vi "Host Datalog.vi"(6 "Operation":enum16{"Create", "Write", "Close", "Header"}(ring)=enum."Write", 8 "error in":errorcluster, 10 "Enable":bool) -> (0 "error out":errorcluster, 5 "datalog Q":refnum<queue>)   [LabVIEW 2021]
doc: "Host data logging is done as four files as Power& Battery, Navigation and HSSS, Ballast and Thrusters, 50KWh battery. every one hour the new files will be created . The data for the vi will be accumulated from Update GUI through Queue"
uses:
  <vilib>/Utility/sysdir.llb/System Directory Type.ctl
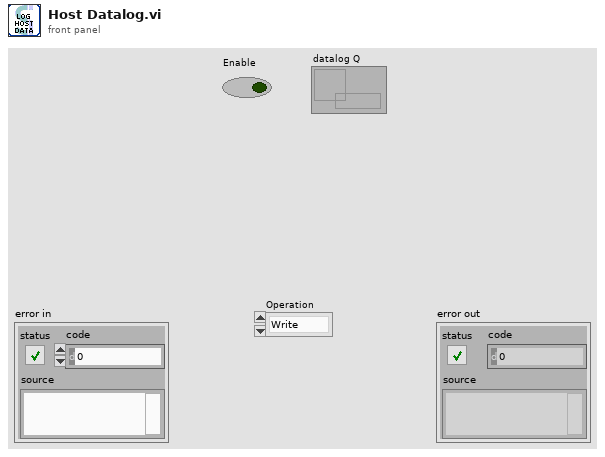
[diagram p1: front panel]
types:
  T1 = enum16{"open", "replace", "create", "open or create", "replace or create", "replace or create with confirmation"}
  T2 = typedef "System Directory Type.ctl" = i32
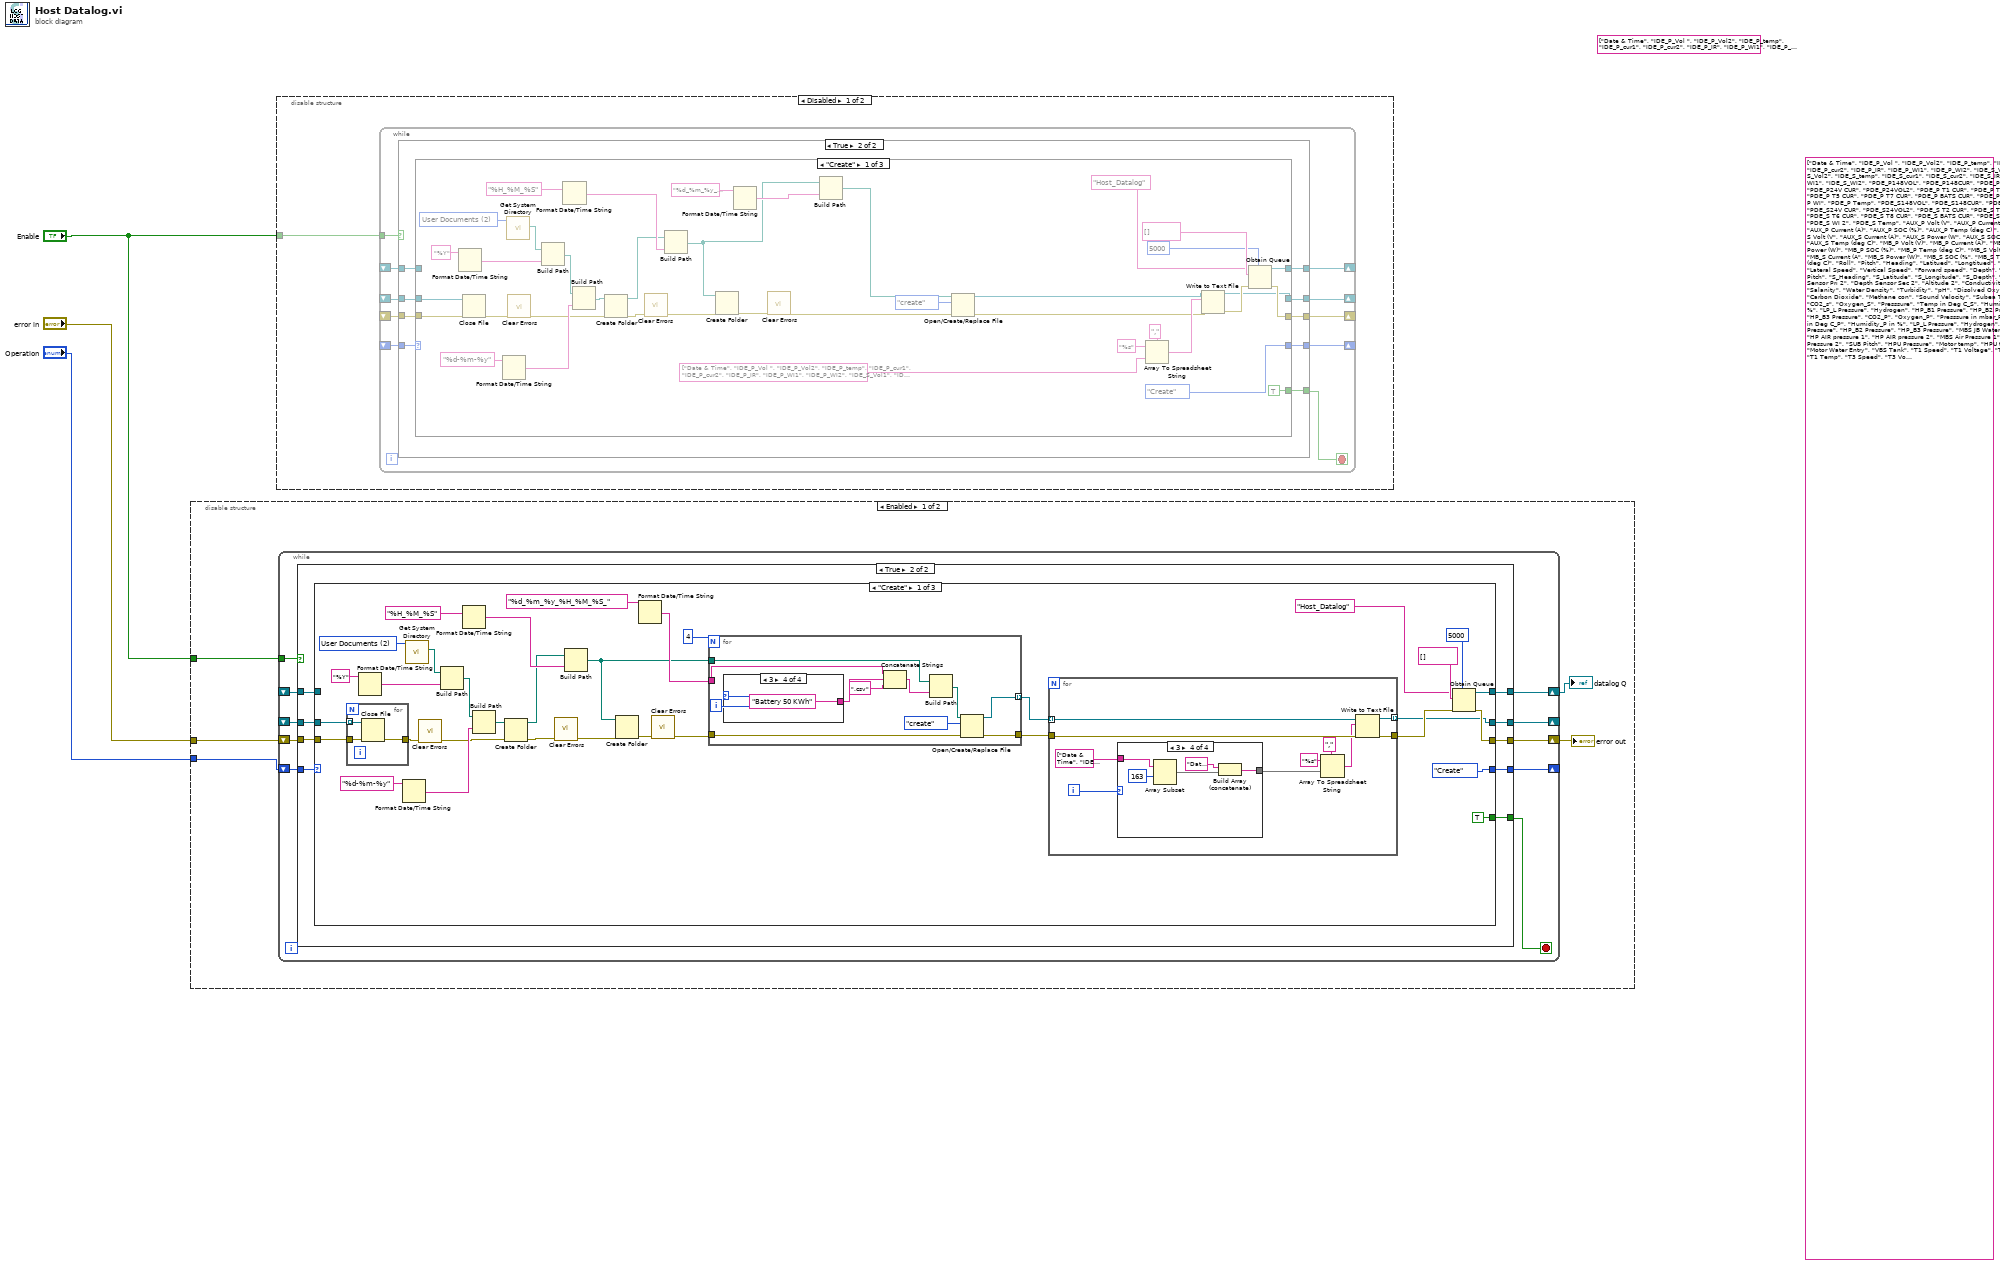
[diagram p0: block diagram]
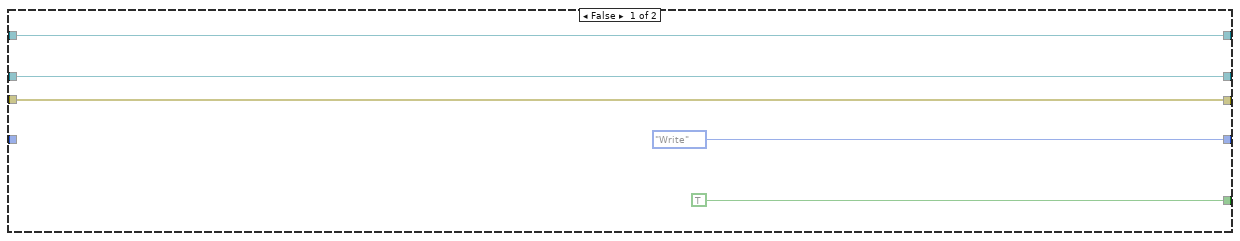
[diagram p2: hidden frame]
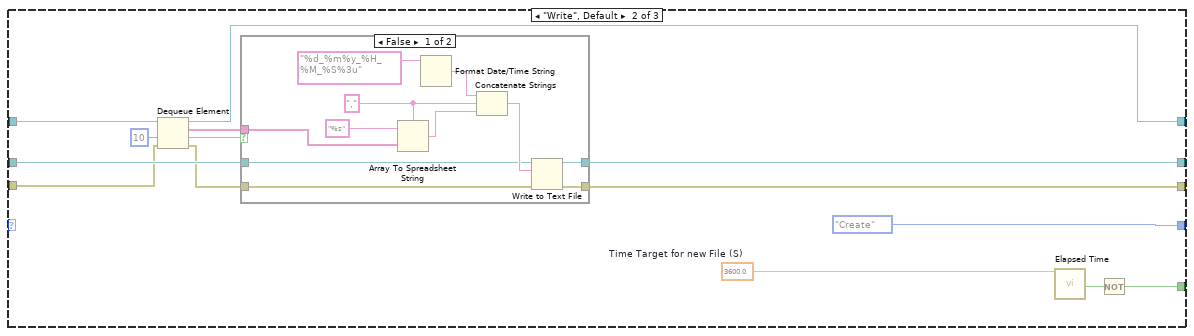
[diagram p3: hidden frame]
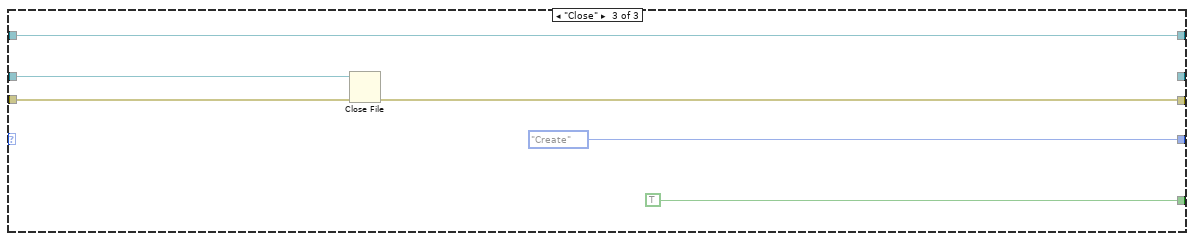
[diagram p5: hidden frame]
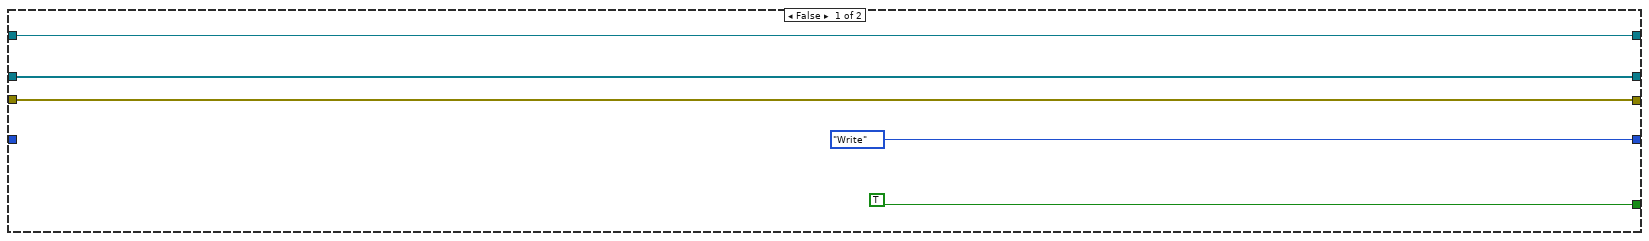
[diagram p7: hidden frame]
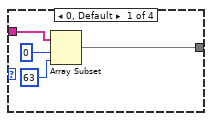
[diagram p8: hidden frame]
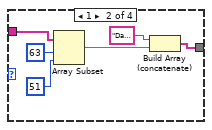
[diagram p9: hidden frame]
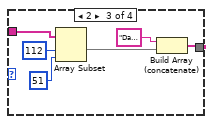
[diagram p10: hidden frame]
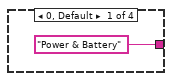
[diagram p11: hidden frame]
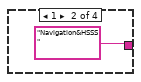
[diagram p12: hidden frame]
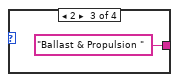
[diagram p13: hidden frame]
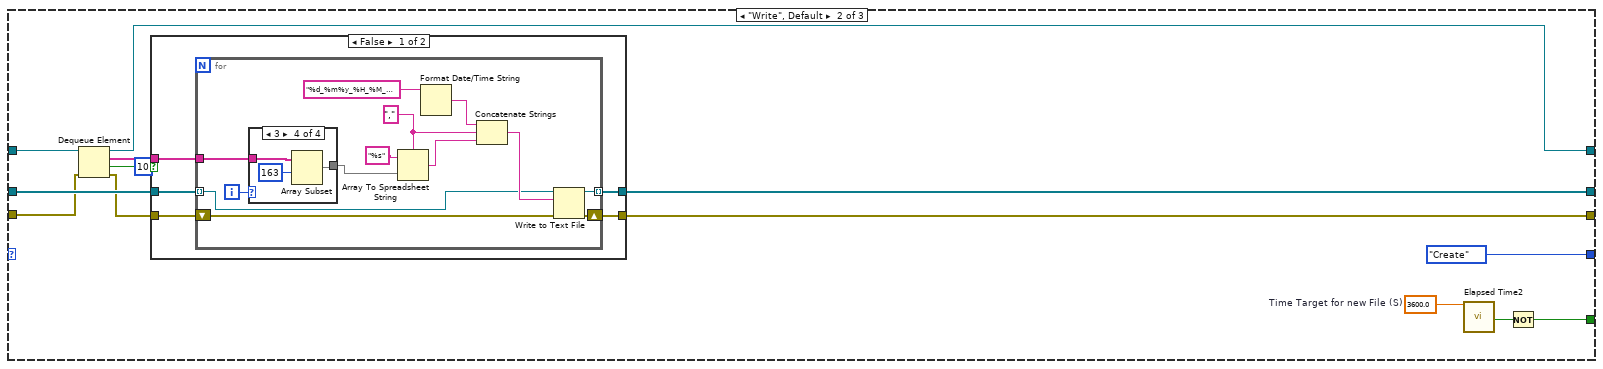
[diagram p14: hidden frame]
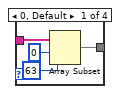
[diagram p15: hidden frame]
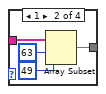
[diagram p16: hidden frame]
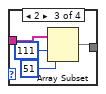
[diagram p17: hidden frame]
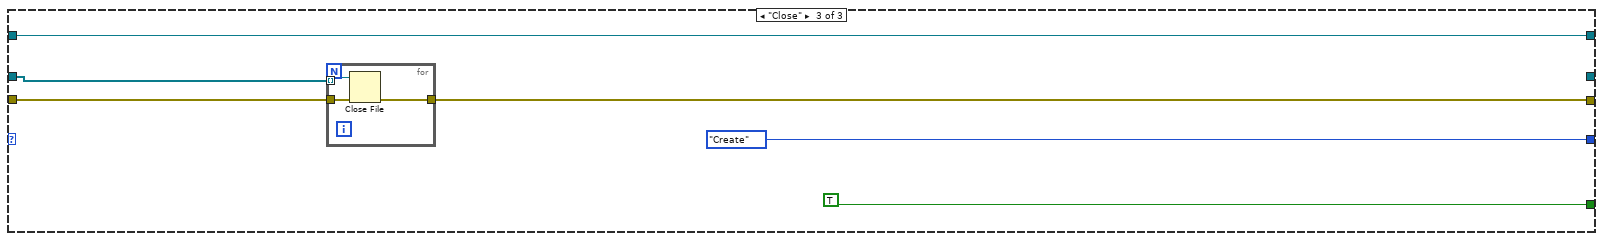
[diagram p19: hidden frame]
diagram:
  (unwired) string[] ["Date & Time", "IDE_P_Vol ", "IDE_P_Vol2", "IDE_P_temp", "IDE_P_cur1", "IDE_P_cur2", "IDE_P_IR", "IDE_P_WI1", "IDE_P_WI2", "IDE_S_Vol1", "IDE_S_Vol2", "IDE_S_temp", "IDE_S_cur1", "IDE_S_cur2", "IDE_S_IR", "IDE_S_WI1", "IDE_S_WI2", "PDE_P148VOL", "PDE_P148CUR", "PDE_P24VOL1", "PDE_P24V CUR", "PDE_P24VOL2", "PDE_P T1 CUR", "PDE_P T3 CUR", "PDE_P T5 CUR", "PDE_P T7 CUR", "PDE_P BATS CUR", "PDE_P WI", "PDE_P WI", "PDE_P Temp", "PDE_S148VOL", "PDE_S148CUR", "PDE_S24VOL1", "PDE_S24V CUR", "PDE_S24VOL2", "PDE_S T2 CUR", "PDE_S T4 CUR", "PDE_S T6 CUR", "PDE_S T8 CUR", "PDE_S BATS CUR", "PDE_S WI 1", "PDE_S WI 2", "PDE_S Temp", "AUX_P Volt (V", "AUX_P Current (A)", "AUX_P Current (A)", "AUX_P SOC (%)", "AUX_P Temp (deg C) ", "AUX_S Volt (V", "AUX_S Current (A)", "AUX_S Power (W", "AUX_S SOC (%)", "AUX_S Temp (deg C)", "MB_P Volt (V)", "MB_P Current (A)", "MB_P Power (W)", "MB_P SOC (%)", "MB_P Temp (deg C)", "MB_S Volt (V)", "MB_S Current (A", "MB_S Power (W)", "MB_S SOC (%", "MB_S Temp (deg C)", "Roll", "Pitch", "Heading", "Latitued", "Longtitued", "Alititued", "Lateral Speed", "Vertical Speed", "Forward speed", "Depth", "S_Roll", "S_Pitch", "S_Heading", "S_Latitude", "S_Longitude", "S_Depth", "Depth Sensor Pri 2", "Depth Sensor Sec 2", "Altitude 2", "Conductivity", "Salanity", "Water Density", "Turbidity", "pH", "Disolved Oxygen", "Carbon Dioxide", "Methane con", "Sound Velocity", "Subea Temp_2", "CO2_s", "Oxygen_S", "Presssure", "Temp in Deg C_S", "Humidity_S in %", "LP_L Pressure", "Hydrogen", "HP_B1 Pressure", "HP_B2 Pressure", "HP_B3 Pressure", "CO2_P", "Oxygen_P", "Presssure in mbar_P", "Temp in Deg C_P", "Humidity_P in %", "LP_L Pressure", "Hydrogen", "HP_B1 Pressure", "HP_B2 Pressure", "HP_B3 Pressure", "MBS JB Water Entry ", "HP AIR pressure 1", "HP AIR pressure 2", "MBS Air Pressure 1", "MBS Air Pressure 2", "SUB Pitch", "HPU Pressure", "Motor temp", "HPU temp", "Motor Water Entry", "VBS Tank", "T1 Speed", "T1 Voltage", "T1 Current", "T1 Temp", "T3 Speed", "T3 Voltage", "T3 Current", "T3 Temp", "T5 Speed", "T5 Voltage", "T5 Current", "T5 Temp", "T7 Speed", "T7 Voltage", "T7 Curren", "T7 Temp", "T2 Speed", "T2 Voltage", "T2 Curren", "T2 Temp", "T4 Speed", "T4 Voltage", "T4 Current", "T4 Temp", "T6 Speed", "T6 Voltage", "T6 Current", "T6 Temp", "T8 Speed", "T8 Voltage", "T8 Current", "T8 Temp", "T1 ctrl", "T3 ctrl", "T5 ctrl", "T7 ctrl", "T2 ctrl", "T4 ctrl", "T6 ctrl", "T8 ctrl", "Current_1", "Voltage_1", "ID Cell Max_1", "Max Temp_1", "ID Cell Min _1", "Min Temp_1", "Temp_1", "SOC_1", "SOH_1", "Current_2", "Voltage_2", "ID Cell Max_2", "Max Temp_2", "ID Cell Min _2", "Min Temp_2", "Temp_2", "SOC_2", "SOH_2", "Current_3", "Voltage_3", "ID Cell Max_3", "Max Temp_3", "ID Cell Min _3", "Min Temp_3", "Temp_3", "SOC_3", "SOH_3", "Current_4", "Voltage_4", "ID Cell Max_4", "Max Temp_4", "ID Cell Min _4", "Min Temp_4", "Temp_4", "SOC_4", "SOH_4", "Current_5", "Voltage_5", "ID Cell Max_5", "Max Temp_5", "ID Cell Min _5", "Min Temp_5", "Temp_5", "SOC_5", "SOH_5", "Current_6", "Voltage_6", "ID Cell Max_6", "Max Temp_6", "ID Cell Min _6", "Min Temp_6", "Temp_6", "SOC_6", "SOH_6", "Current_7", "Voltage_7", "ID Cell Max_7", "Max Temp_7", "ID Cell Min _7", "Min Temp_7", "Temp_7", "SOC_7", "SOH_7", "Current_8", "Voltage_8", "ID Cell Max_8", "Max Temp_8", "ID Cell Min _8", "Min Temp_8", "Temp_8", "SOC_8", "SOH_8", "Current_9", "Voltage_9", "ID Cell Max_9", "Max Temp_9", "ID Cell Min _9", "Min Temp_9", "Temp_9", "SOC_9", "SOH_9", "Current_10", "Voltage_10", "ID Cell Max_10", "Max Temp_10", "ID Cell Min _10", "Min Temp_10", "Temp_10", "SOC_10", "SOH_10", "BAT VOL", "BAT TEMP", "BAT SOC", "BAT CUR", "BAT VOL 2", "BAT TEMP 2", "BAT SOC 2", "BAT CUR 2"]
  (unwired) string[] ["Date & Time", "IDE_P_Vol ", "IDE_P_Vol2", "IDE_P_temp", "IDE_P_cur1", "IDE_P_cur2", "IDE_P_IR", "IDE_P_WI1", "IDE_P_WI2", "IDE_S_Vol1", "IDE_S_Vol2", "IDE_S_temp", "IDE_S_cur1", "IDE_S_cur2", "IDE_S_IR", "IDE_S_WI1", "IDE_S_WI2", "PDE_P148VOL", "PDE_P148CUR", "PDE_P24VOL1", "PDE_P24V CUR", "PDE_P24VOL2", "PDE_P T1 CUR", "PDE_P T3 CUR", "PDE_P T5 CUR", "PDE_P T7 CUR", "PDE_P BATS CUR", "PDE_P WI", "PDE_P WI", "PDE_P Temp", "PDE_S148VOL", "PDE_S148CUR", "PDE_S24VOL1", "PDE_S24V CUR", "PDE_S24VOL2", "PDE_S T1 CUR", "PDE_S T3 CUR", "PDE_S T5 CUR", "PDE_S T7 CUR", "PDE_S BATS CUR", "PDE_S WI 1", "PDE_S WI 2", "PDE_S Temp"]
  n1 = disable-structure shown="Enabled" {
    disable-tunnel: "Enable" -> [w8 _]
    disable-tunnel: "error in" -> [w7 _]
    disable-tunnel: "Operation" -> [w6 _]
    frame Enabled {
      n2 = while {
        shift-right: [w17] -> _
        shift-left: _ -> [w16]
        shift-right: [w15] -> w4
        shift-left: w7 -> [w14]
        shift-right: [w12] -> _
        shift-left: w6 -> [w18]
        shift-right: [w11] -> w5
        shift-left: _ -> [w10]
        tunnel: w8 -> [w9]
        stop <- w13 stop-if-true
        n3 = case shown="True" w9 {
          tunnel: w18 -> [_ w32]
          tunnel: [w23 w31] -> w17
          tunnel: w16 -> [w23 w30]
          tunnel: [w22 w29] -> w15
          tunnel: w14 -> [w22 w28]
          tunnel: [TRUE w27] -> w13
          tunnel: [enum16{"Create", "Write", "Close"}."Write" ("Operation 2") w26] -> w12
          tunnel: [w19 w25] -> w11
          tunnel: w10 -> [w19 w24]
          frame False {
          }
          frame True {
            n4 = case shown="\"Create\"" w32 {
              tunnel: [w44 w127 _] -> w31
              tunnel: w30 -> [w36 w129 w165]
              tunnel: [w50 w128 w169] -> w29
              tunnel: w28 -> [w55 w122 w170]
              tunnel: [TRUE w125 TRUE] -> w27
              tunnel: [enum16{"Create", "Write", "Close", "Header"}."Create" ("Operation") enum16{"Create", "Write", "Close", "Header"}."Create" ("Operation") enum16{"Create", "Write", "Close", "Header"}."Create" ("Operation")] -> w26
              tunnel: [w48 w118 w167] -> w25
              tunnel: w24 -> [_ w123 w167]
              frame "Create" {
                w66 = T2 2 items=["User Home"=0, "User Desktop"=1, "User Documents"=2, "User Application Data"=3, "User Preferences"=4, "User Temporary"=5, "Public Documents"=6, "Public Application Data"=7, "Public Preferences"=8, "Public Cache"=13, "System Core Libraries"=9, "System Installed Libraries"=10, "Application Files"=11, "Boot Volume Root"=12] ("system directory type")
                n5 = for {
                  tunnel: w55 -> [w69]
                  tunnel: [w68] -> w54
                  tunnel: w36 -> [w67] mode=indexing
                  n6 = Close File(refnum=w67, error in=w69) -> (error out=w68:errorcluster)  [unwired: 1 out]
                }
                n7 = Format Date/Time String(time format string (%c)="%Y") -> (date/time string=w62:string)  [unwired: 2 in]
                n8 = Format Date/Time String(time format string (%c)="%d-%m-%y") -> (date/time string=w60:string)  [unwired: 2 in]
                n9 = call <vilib>:"Get System Directory.vi"("system directory type"=w66) -> ("system directory"=w63:path)  [unwired: 10 in]
                n10 = call <vilib>:"Clear Errors.vi"("error in (no error)"=w54) -> ("error out"=w53:errorcluster)  [unwired: 5 in, 1 out]
                n11 = Build Path(base path=w63, name or relative path=w62) -> (appended path=w61:path)
                n12 = Format Date/Time String(time format string (%c)="%H_%M_%S") -> (date/time string=w41:string)  [unwired: 2 in]
                n13 = Build Path(base path=w61, name or relative path=w60) -> (appended path=w57:path)
                n14 = Create Folder(path (use dialog)=w57, error in=w53) -> (created path=w39:path, error out=w43:errorcluster)  [unwired: 1 in, 1 out]
                n15 = call <vilib>:"Clear Errors.vi"("error in (no error)"=w43) -> ("error out"=w42:errorcluster)  [unwired: 5 in, 1 out]
                n16 = Build Path(base path=w39, name or relative path=w41) -> (appended path=w33:path)
                n17 = Create Folder(path (use dialog)=w33, error in=w42) -> (error out=w38:errorcluster)  [unwired: 1 in, 2 out]
                n18 = Format Date/Time String(time format string (%c)="%d_%m_%y_%H_%M_%S_") -> (date/time string=w34:string)  [unwired: 2 in]
                n19 = call <vilib>:"Clear Errors.vi"("error in (no error)"=w38) -> ("error out"=w58:errorcluster)  [unwired: 5 in, 1 out]
                n20 = for {
                  N: 4 -> [_]
                  tunnel: [w108] -> w37 mode=indexing
                  tunnel: w34 -> [w105]
                  tunnel: w33 -> [w104]
                  tunnel: w58 -> [w110]
                  tunnel: [w109] -> w46
                  i -> [w102]
                  n21 = case shown="3" w102 {
                    tunnel: ["Power & Battery" ("type") "Navigation&HSSS" ("type") "Ballast & Propulsion " ("type") "Battery 50 KWh" ("type")] -> w101
                    frame 0, Default {
                    }
                    frame 1 {
                    }
                    frame 2 {
                    }
                    frame 3 {
                    }
                  }
                  n22 = Concatenate Strings(w105, w101, ".csv" ("type")) -> (w106:string)
                  n23 = Build Path(base path=w104, name or relative path=w106) -> (appended path=w103:path)
                  n24 = Open/Create/Replace File(file path (use dialog)=w103, error in=w110, operation (0:open)=T1."create") -> (refnum out=w108:refnum<file>, error out=w109:errorcluster)  [unwired: 3 in, 1 out]
                }
                n25 = for {
                  tunnel: w37 -> [w77] mode=indexing
                  tunnel: [w76] -> w44 mode=indexing
                  tunnel: w46 -> [w79]
                  tunnel: [w78] -> w45
                  i -> [w73]
                  n26 = case shown="3" w73 {
                    tunnel: string[] ["Date & Time", "IDE_P_Vol ", "IDE_P_Vol2", "IDE_P_temp", "IDE_P_cur1", "IDE_P_cur2", "IDE_P_IR", "IDE_P_WI1", "IDE_P_WI2", "IDE_S_Vol1", "IDE_S_Vol2", "IDE_S_temp", "IDE_S_cur1", "IDE_S_cur2", "IDE_S_IR", "IDE_S_WI1", "IDE_S_WI2", "PDE_P148VOL", "PDE_P148CUR", "PDE_P24VOL1", "PDE_P24V CUR", "PDE_P24VOL2", "PDE_P T1 CUR", "PDE_P T3 CUR", "PDE_P T5 CUR", "PDE_P T7 CUR", "PDE_P BATS CUR", "PDE_P WI", "PDE_P WI", "PDE_P Temp", "PDE_S148VOL", "PDE_S148CUR", "PDE_S24VOL1", "PDE_S24V CUR", "PDE_S24VOL2", "PDE_S T2 CUR", "PDE_S T4 CUR", "PDE_S T6 CUR", "PDE_S T8 CUR", "PDE_S BATS CUR", "PDE_S WI 1", "PDE_S WI 2", "PDE_S Temp", "AUX_P Volt (V", "AUX_P Current (A)", "AUX_P Current (A)", "AUX_P SOC (%)", "AUX_P Temp (deg C) ", "AUX_S Volt (V", "AUX_S Current (A)", "AUX_S Power (W", "AUX_S SOC (%)", "AUX_S Temp (deg C)", "MB_P Volt (V)", "MB_P Current (A)", "MB_P Power (W)", "MB_P SOC (%)", "MB_P Temp (deg C)", "MB_S Volt (V)", "MB_S Current (A", "MB_S Power (W)", "MB_S SOC (%", "MB_S Temp (deg C)", "Roll", "Pitch", "Heading", "Latitued", "Longtitued", "Alititued", "Lateral Speed", "Vertical Speed", "Forward speed", "Depth", "S_Roll", "S_Pitch", "S_Heading", "S_Latitude", "S_Longitude", "S_Depth", "Depth Sensor Pri 2", "Depth Sensor Sec 2", "Altitude 2", "Conductivity", "Salanity", "Water Density", "Turbidity", "pH", "Disolved Oxygen", "Carbon Dioxide", "Methane con", "Sound Velocity", "Subea Temp_2", "CO2_s", "Oxygen_S", "Presssure", "Temp in Deg C_S", "Humidity_S in %", "LP_L Pressure", "Hydrogen", "HP_B1 Pressure", "HP_B2 Pressure", "HP_B3 Pressure", "CO2_P", "Oxygen_P", "Presssure in mbar_P", "Temp in Deg C_P", "Humidity_P in %", "LP_L Pressure", "Hydrogen", "HP_B1 Pressure", "HP_B2 Pressure", "HP_B3 Pressure", "MBS JB Water Entry ", "HP AIR pressure 1", "HP AIR pressure 2", "MBS Air Pressure 1", "MBS Air Pressure 2", "SUB Pitch", "HPU Pressure", "Motor temp", "HPU temp", "Motor Water Entry", "VBS Tank", "T1 Speed", "T1 Voltage", "T1 Current", "T1 Temp", "T3 Speed", "T3 Voltage", "T3 Current", "T3 Temp", "T5 Speed", "T5 Voltage", "T5 Current", "T5 Temp", "T7 Speed", "T7 Voltage", "T7 Curren", "T7 Temp", "T2 Speed", "T2 Voltage", "T2 Curren", "T2 Temp", "T4 Speed", "T4 Voltage", "T4 Current", "T4 Temp", "T6 Speed", "T6 Voltage", "T6 Current", "T6 Temp", "T8 Speed", "T8 Voltage", "T8 Current", "T8 Temp", "T1 ctrl", "T3 ctrl", "T5 ctrl", "T7 ctrl", "T2 ctrl", "T4 ctrl", "T6 ctrl", "T8 ctrl", "Current_1", "Voltage_1", "ID Cell Max_1", "Max Temp_1", "ID Cell Min _1", "Min Temp_1", "Temp_1", "SOC_1", "SOH_1", "Current_2", "Voltage_2", "ID Cell Max_2", "Max Temp_2", "ID Cell Min _2", "Min Temp_2", "Temp_2", "SOC_2", "SOH_2", "Current_3", "Voltage_3", "ID Cell Max_3", "Max Temp_3", "ID Cell Min _3", "Min Temp_3", "Temp_3", "SOC_3", "SOH_3", "Current_4", "Voltage_4", "ID Cell Max_4", "Max Temp_4", "ID Cell Min _4", "Min Temp_4", "Temp_4", "SOC_4", "SOH_4", "Current_5", "Voltage_5", "ID Cell Max_5", "Max Temp_5", "ID Cell Min _5", "Min Temp_5", "Temp_5", "SOC_5", "SOH_5", "Current_6", "Voltage_6", "ID Cell Max_6", "Max Temp_6", "ID Cell Min _6", "Min Temp_6", "Temp_6", "SOC_6", "SOH_6", "Current_7", "Voltage_7", "ID Cell Max_7", "Max Temp_7", "ID Cell Min _7", "Min Temp_7", "Temp_7", "SOC_7", "SOH_7", "Current_8", "Voltage_8", "ID Cell Max_8", "Max Temp_8", "ID Cell Min _8", "Min Temp_8", "Temp_8", "SOC_8", "SOH_8", "Current_9", "Voltage_9", "ID Cell Max_9", "Max Temp_9", "ID Cell Min _9", "Min Temp_9", "Temp_9", "SOC_9", "SOH_9", "Current_10", "Voltage_10", "ID Cell Max_10", "Max Temp_10", "ID Cell Min _10", "Min Temp_10", "Temp_10", "SOC_10", "SOH_10", "BAT VOL", "BAT TEMP", "BAT SOC", "BAT CUR", "BAT VOL 2", "BAT TEMP 2", "BAT SOC 2", "BAT CUR 2", "altimeter", "DO", "SUB SEA TEMP", "PDE_S VOLTAGE", "PDE_S CURRENT", "PDE_S TEMP", "PDE_S IR", "IDE_S VOLTAGE 1", "IDE_S CURRENT", "IDE_S TEMP", "IDE_S IR", "T2 VOLTAGE", "T2 CURRENT", "T2 SPEED", "T2 C TEMP", "T2 HS TEMP", "T2 W TEMP", "T4 VOLTAGE", "T4 CURRENT", "T4 SPEED", "T4 C TEMP", "T4 HS TEMP", "T4 W TEMP", "T6 VOLTAGE", "T6 CURRENT", "T6 SPEED", "T6 C TEMP", "T6 HS TEMP", "T6 W TEMP", "T8 VOLTAGE", "T8 CURRENT", "T8 SPEED", "T8 C TEMP", "T8 HS TEMP", "T8 W TEMP"] ("Array") -> [w81 w87 w93 w99]
                    tunnel: [w80 w85 w91 w96] -> w71
                    frame 0, Default {
                      n27 = Array Subset(array=w81, index=0, length=63) -> (w80:string[])
                    }
                    frame 1 {
                      n28 = Array Subset(array=w87, index=63, length=51) -> (w86:string[])
                      n29 = Build Array (concatenate)("Date & Time", w86) -> (w85:string[])
                    }
                    frame 2 {
                      n30 = Array Subset(array=w93, index=112, length=51) -> (w92:string[])
                      n31 = Build Array (concatenate)("Date & Time", w92) -> (w91:string[])
                    }
                    frame 3 {
                      n32 = Array Subset(array=w99, index=163) -> (w97:string[])  [unwired: 1 in]
                      n33 = Build Array (concatenate)("Date & Time", w97) -> (w96:string[])
                    }
                  }
                  n34 = Array To Spreadsheet String(delimiter (Tab)=",", array=w71, 3:"%s" ("format string")) -> (spreadsheet string=w70:string)
                  n35 = Write to Text File(file (use dialog)=w77, text=w70, error in=w79) -> (refnum out=w76:refnum<file>, error out=w78:errorcluster)  [unwired: 1 in, 1 out]
                }
                n36 = Obtain Queue(max queue size (-1, unlimited)=5000, name (unnamed)="Host_Datalog", element data type=string[] [] ("Data in"), error in (no error)=w45) -> (queue out=w48:refnum<queue>, error out=w50:errorcluster)  [unwired: 1 in, 1 out]
              }
              frame "Write", Default {
                w124 = 3600.0  # Time Target for new File (S)
                n37 = Dequeue Element(queue=w123, timeout in ms (-1)=10, error in (no error)=w122) -> (queue out=w118:refnum<queue>, element=w119:string[], timed out?=w120:bool, error out=w121:errorcluster)
                n38 = case shown="False" w120 {
                  tunnel: w129 -> [w130 w164]
                  tunnel: [w134 w163] -> w128
                  tunnel: [w131 w164] -> w127
                  tunnel: w121 -> [w133 w163]
                  tunnel: w119 -> [w132 _]
                  frame False {
                    n39 = for {
                      tunnel: w132 -> [w138]
                      tunnel: [w139] -> w131 mode=indexing
                      shift-right: [w142] -> w134
                      shift-left: w133 -> [w140]
                      tunnel: w130 -> [w135] mode=indexing
                      i -> [w136]
                      w143 = "," ("delimiter (Tab)")
                      n40 = case shown="3" w136 {
                        tunnel: [w149 w153 w157 w161] -> w137
                        tunnel: w138 -> [w148 w152 w156 w160]
                        frame 0, Default {
                          n41 = Array Subset(array=w148, index=0, length=63) -> (w149:string[])
                        }
                        frame 1 {
                          n42 = Array Subset(array=w152, index=63, length=49) -> (w153:string[])
                        }
                        frame 2 {
                          n43 = Array Subset(array=w156, index=111, length=51) -> (w157:string[])
                        }
                        frame 3 {
                          n44 = Array Subset(array=w160, index=163) -> (w161:string[])  [unwired: 1 in]
                        }
                      }
                      n45 = Array To Spreadsheet String(delimiter (Tab)=w143, array=w137, 3:"%s" ("format string")) -> (spreadsheet string=w141:string)
                      n46 = Format Date/Time String(time format string (%c)="%d_%m%y_%H_%M_%S%3u") -> (date/time string=w146:string)  [unwired: 2 in]
                      n47 = Concatenate Strings(w146, w143, w141) -> (w147:string)
                      n48 = Write to Text File(file (use dialog)=w135, text=w147, error in=w140) -> (refnum out=w139:refnum<file>, error out=w142:errorcluster)  [unwired: 1 in, 1 out]
                    }
                  }
                  frame True {
                  }
                }
                n49 = call "Elapsed Time2"("Time Target (s)"=w124) -> ("Time has Elapsed"=w126:bool)  [unwired: 11 in, 7 out]
                n50 = Not(x=w126) -> (.not. x?=w125:bool)
              }
              frame "Close" {
                n51 = for {
                  tunnel: w170 -> [w173]
                  tunnel: [w172] -> w169
                  tunnel: w165 -> [w171] mode=indexing
                  n52 = Close File(refnum=w171, error in=w173) -> (error out=w172:errorcluster)  [unwired: 1 out]
                }
              }
            }
          }
        }
      }
      "error out" <- w4
      "datalog Q" <- w5
    }
    frame Disabled {
    }
  }
  n53 = disable-structure shown="Disabled" {
    disable-tunnel: "Enable" -> [w176 _]
    frame Disabled {
      n54 = while {
        shift-right: [w185] -> _
        shift-left: _ -> [w184]
        shift-right: [w183] -> _
        shift-left: [w182] -> w174
        tunnel: w176 -> [w181]
        shift-right: [w179] -> _
        shift-left: [w186] -> w175
        shift-right: [w178] -> _
        shift-left: _ -> [w177]
        stop <- w180 stop-if-true
        n55 = case shown="True" w181 {
          tunnel: w186 -> [_ w200]
          tunnel: [w191 w199] -> w185
          tunnel: w184 -> [w191 w198]
          tunnel: [w190 w197] -> w183
          tunnel: w182 -> [w190 w196]
          tunnel: [TRUE w195] -> w180
          tunnel: [enum16{"Create", "Write", "Close"}."Write" ("Operation 2") w194] -> w179
          tunnel: [w187 w193] -> w178
          tunnel: w177 -> [w187 w192]
          frame False {
          }
          frame True {
            n56 = case shown="\"Create\"" w200 {
              tunnel: [w209 w251 _] -> w199
              tunnel: w198 -> [w223 w253 w270]
              tunnel: [w219 w252 w271] -> w197
              tunnel: w196 -> [w225 w246 w272]
              tunnel: [TRUE w249 TRUE] -> w195
              tunnel: [enum16{"Create", "Write", "Close", "Header"}."Create" ("Operation") enum16{"Create", "Write", "Close", "Header"}."Create" ("Operation") enum16{"Create", "Write", "Close", "Header"}."Create" ("Operation")] -> w194
              tunnel: [w217 w242 w268] -> w193
              tunnel: w192 -> [_ w247 w268]
              frame "Create" {
                w239 = T2 2 items=["User Home"=0, "User Desktop"=1, "User Documents"=2, "User Application Data"=3, "User Preferences"=4, "User Temporary"=5, "Public Documents"=6, "Public Application Data"=7, "Public Preferences"=8, "Public Cache"=13, "System Core Libraries"=9, "System Installed Libraries"=10, "Application Files"=11, "Boot Volume Root"=12] ("system directory type")
                n57 = Format Date/Time String(time format string (%c)="%Y") -> (date/time string=w235:string)  [unwired: 2 in]
                n58 = Close File(refnum=w223, error in=w225) -> (error out=w224:errorcluster)  [unwired: 1 out]
                n59 = Format Date/Time String(time format string (%c)="%d-%m-%y") -> (date/time string=w233:string)  [unwired: 2 in]
                n60 = call <vilib>:"Get System Directory.vi"("system directory type"=w239) -> ("system directory"=w236:path)  [unwired: 10 in]
                n61 = call <vilib>:"Clear Errors.vi"("error in (no error)"=w224) -> ("error out"=w222:errorcluster)  [unwired: 5 in, 1 out]
                n62 = Build Path(base path=w236, name or relative path=w235) -> (appended path=w234:path)
                n63 = Format Date/Time String(time format string (%c)="%H_%M_%S") -> (date/time string=w205:string)  [unwired: 2 in]
                n64 = Build Path(base path=w234, name or relative path=w233) -> (appended path=w227:path)
                n65 = Create Folder(path (use dialog)=w227, error in=w222) -> (created path=w202:path, error out=w207:errorcluster)  [unwired: 1 in, 1 out]
                n66 = call <vilib>:"Clear Errors.vi"("error in (no error)"=w207) -> ("error out"=w206:errorcluster)  [unwired: 5 in, 1 out]
                n67 = Build Path(base path=w202, name or relative path=w205) -> (appended path=w203:path)
                n68 = Create Folder(path (use dialog)=w203, error in=w206) -> (error out=w201:errorcluster)  [unwired: 1 in, 2 out]
                n69 = Format Date/Time String(time format string (%c)="%d_%m_%y_%H_%M_%S.csv") -> (date/time string=w231:string)  [unwired: 2 in]
                n70 = call <vilib>:"Clear Errors.vi"("error in (no error)"=w201) -> ("error out"=w228:errorcluster)  [unwired: 5 in, 1 out]
                n71 = Build Path(base path=w203, name or relative path=w231) -> (appended path=w229:path)
                n72 = Open/Create/Replace File(file path (use dialog)=w229, error in=w228, operation (0:open)=T1."create") -> (refnum out=w210:refnum<file>, error out=w212:errorcluster)  [unwired: 3 in, 1 out]
                n73 = Array To Spreadsheet String(delimiter (Tab)=",", array=string[] ["Date & Time", "IDE_P_Vol ", "IDE_P_Vol2", "IDE_P_temp", "IDE_P_cur1", "IDE_P_cur2", "IDE_P_IR", "IDE_P_WI1", "IDE_P_WI2", "IDE_S_Vol1", "IDE_S_Vol2", "IDE_S_temp", "IDE_S_cur1", "IDE_S_cur2", "IDE_S_IR", "IDE_S_WI1", "IDE_S_WI2", "PDE_P148VOL", "PDE_P148CUR", "PDE_P24VOL1", "PDE_P24V CUR", "PDE_P24VOL2", "PDE_P T1 CUR", "PDE_P T3 CUR", "PDE_P T5 CUR", "PDE_P T7 CUR", "PDE_P BATS CUR", "PDE_P WI", "PDE_P WI", "PDE_P Temp", "PDE_S148VOL", "PDE_S148CUR", "PDE_S24VOL1", "PDE_S24V CUR", "PDE_S24VOL2", "PDE_S T2 CUR", "PDE_S T4 CUR", "PDE_S T6 CUR", "PDE_S T8 CUR", "PDE_S BATS CUR", "PDE_S WI 1", "PDE_S WI 2", "PDE_S Temp", "AUX_P Volt (V", "AUX_P Current (A)", "AUX_P Current (A)", "AUX_P SOC (%)", "AUX_P Temp (deg C) ", "AUX_S Volt (V", "AUX_S Current (A)", "AUX_S Power (W", "AUX_S SOC (%)", "AUX_S Temp (deg C)", "MB_P Volt (V)", "MB_P Current (A)", "MB_P Power (W)", "MB_P SOC (%)", "MB_P Temp (deg C)", "MB_S Volt (V)", "MB_S Current (A", "MB_S Power (W)", "MB_S SOC (%", "MB_S Temp (deg C)", "Roll", "Pitch", "Heading", "Latitued", "Longtitued", "Alititued", "Lateral Speed", "Vertical Speed", "Forward speed", "Depth", "S_Roll", "S_Pitch", "S_Heading", "S_Latitude", "S_Longitude", "S_Depth", "Depth Sensor Pri 2", "Depth Sensor Sec 2", "Altitude 2", "Conductivity", "Salanity", "Water Density", "Turbidity", "pH", "Disolved Oxygen", "Carbon Dioxide", "Methane con", "Sound Velocity", "Subea Temp_2", "CO2_s", "Oxygen_S", "Presssure", "Temp in Deg C_S", "Humidity_S in %", "LP_L Pressure", "Hydrogen", "HP_B1 Pressure", "HP_B2 Pressure", "HP_B3 Pressure", "CO2_P", "Oxygen_P", "Presssure in mbar_P", "Temp in Deg C_P", "Humidity_P in %", "LP_L Pressure", "Hydrogen", "HP_B1 Pressure", "HP_B2 Pressure", "HP_B3 Pressure", "MBS JB Water Entry ", "HP AIR pressure 1", "HP AIR pressure 2", "MBS Air Pressure 1", "MBS Air Pressure 2", "SUB Pitch", "HPU Pressure", "Motor temp", "HPU temp", "Motor Water Entry", "VBS Tank", "T1 Speed", "T1 Voltage", "T1 Current", "T1 Temp", "T3 Speed", "T3 Voltage", "T3 Current", "T3 Temp", "T5 Speed", "T5 Voltage", "T5 Current", "T5 Temp", "T7 Speed", "T7 Voltage", "T7 Curren", "T7 Temp", "T2 Speed", "T2 Voltage", "T2 Curren", "T2 Temp", "T4 Speed", "T4 Voltage", "T4 Current", "T4 Temp", "T6 Speed", "T6 Voltage", "T6 Current", "T6 Temp", "T8 Speed", "T8 Voltage", "T8 Current", "T8 Temp", "T1 ctrl", "T3 ctrl", "T5 ctrl", "T7 ctrl", "T2 ctrl", "T4 ctrl", "T6 ctrl", "T8 ctrl", "Current_1", "Voltage_1", "ID Cell Max_1", "Max Temp_1", "ID Cell Min _1", "Min Temp_1", "Temp_1", "SOC_1", "SOH_1", "Current_2", "Voltage_2", "ID Cell Max_2", "Max Temp_2", "ID Cell Min _2", "Min Temp_2", "Temp_2", "SOC_2", "SOH_2", "Current_3", "Voltage_3", "ID Cell Max_3", "Max Temp_3", "ID Cell Min _3", "Min Temp_3", "Temp_3", "SOC_3", "SOH_3", "Current_4", "Voltage_4", "ID Cell Max_4", "Max Temp_4", "ID Cell Min _4", "Min Temp_4", "Temp_4", "SOC_4", "SOH_4", "Current_5", "Voltage_5", "ID Cell Max_5", "Max Temp_5", "ID Cell Min _5", "Min Temp_5", "Temp_5", "SOC_5", "SOH_5", "Current_6", "Voltage_6", "ID Cell Max_6", "Max Temp_6", "ID Cell Min _6", "Min Temp_6", "Temp_6", "SOC_6", "SOH_6", "Current_7", "Voltage_7", "ID Cell Max_7", "Max Temp_7", "ID Cell Min _7", "Min Temp_7", "Temp_7", "SOC_7", "SOH_7", "Current_8", "Voltage_8", "ID Cell Max_8", "Max Temp_8", "ID Cell Min _8", "Min Temp_8", "Temp_8", "SOC_8", "SOH_8", "Current_9", "Voltage_9", "ID Cell Max_9", "Max Temp_9", "ID Cell Min _9", "Min Temp_9", "Temp_9", "SOC_9", "SOH_9", "Current_10", "Voltage_10", "ID Cell Max_10", "Max Temp_10", "ID Cell Min _10", "Min Temp_10", "Temp_10", "SOC_10", "SOH_10", "BAT VOL", "BAT TEMP", "BAT SOC", "BAT CUR", "BAT VOL 2", "BAT TEMP 2", "BAT SOC 2", "BAT CUR 2"], 3:"%s" ("format string")) -> (spreadsheet string=w215:string)
                n74 = Write to Text File(file (use dialog)=w210, text=w215, error in=w212) -> (refnum out=w209:refnum<file>, error out=w211:errorcluster)  [unwired: 1 in, 1 out]
                n75 = Obtain Queue(max queue size (-1, unlimited)=5000, name (unnamed)="Host_Datalog", element data type=string[] [] ("Data in"), error in (no error)=w211) -> (queue out=w217:refnum<queue>, error out=w219:errorcluster)  [unwired: 1 in, 1 out]
              }
              frame "Write", Default {
                w248 = 3600.0  # Time Target for new File (S)
                n76 = Dequeue Element(queue=w247, timeout in ms (-1)=10, error in (no error)=w246) -> (queue out=w242:refnum<queue>, element=w243:string[], timed out?=w244:bool, error out=w245:errorcluster)
                n77 = case shown="False" w244 {
                  tunnel: w253 -> [w259 w266]
                  tunnel: [w258 w265] -> w252
                  tunnel: [w257 w266] -> w251
                  tunnel: w245 -> [w255 w265]
                  tunnel: w243 -> [w254 _]
                  frame False {
                    w260 = "," ("delimiter (Tab)")
                    n78 = Array To Spreadsheet String(delimiter (Tab)=w260, array=w254, 3:"%s" ("format string")) -> (spreadsheet string=w256:string)
                    n79 = Format Date/Time String(time format string (%c)="%d_%m%y_%H_%M_%S%3u") -> (date/time string=w263:string)  [unwired: 2 in]
                    n80 = Concatenate Strings(w263, w260, w256) -> (w264:string)
                    n81 = Write to Text File(file (use dialog)=w259, text=w264, error in=w255) -> (refnum out=w257:refnum<file>, error out=w258:errorcluster)  [unwired: 1 in, 1 out]
                  }
                  frame True {
                  }
                }
                n82 = call "Elapsed Time"("Time Target (s)"=w248) -> ("Time has Elapsed"=w250:bool)  [unwired: 11 in, 7 out]
                n83 = Not(x=w250) -> (.not. x?=w249:bool)
              }
              frame "Close" {
                n84 = Close File(refnum=w270, error in=w272) -> (error out=w271:errorcluster)  [unwired: 1 out]
              }
            }
          }
        }
      }
    }
    frame Enabled {
    }
  }
